vi "Button Press Event.vi"(8 "error in (no error)":errorcluster, 9 "Event Time":u32, 10 "Buttons":bool[](array[boolean]), 11 "State Data in":T1) -> (0 "error out":errorcluster, 3 "State Data out":T1)   [LabVIEW 2025]
uses:
  State Data.ctl
  Team.ctl
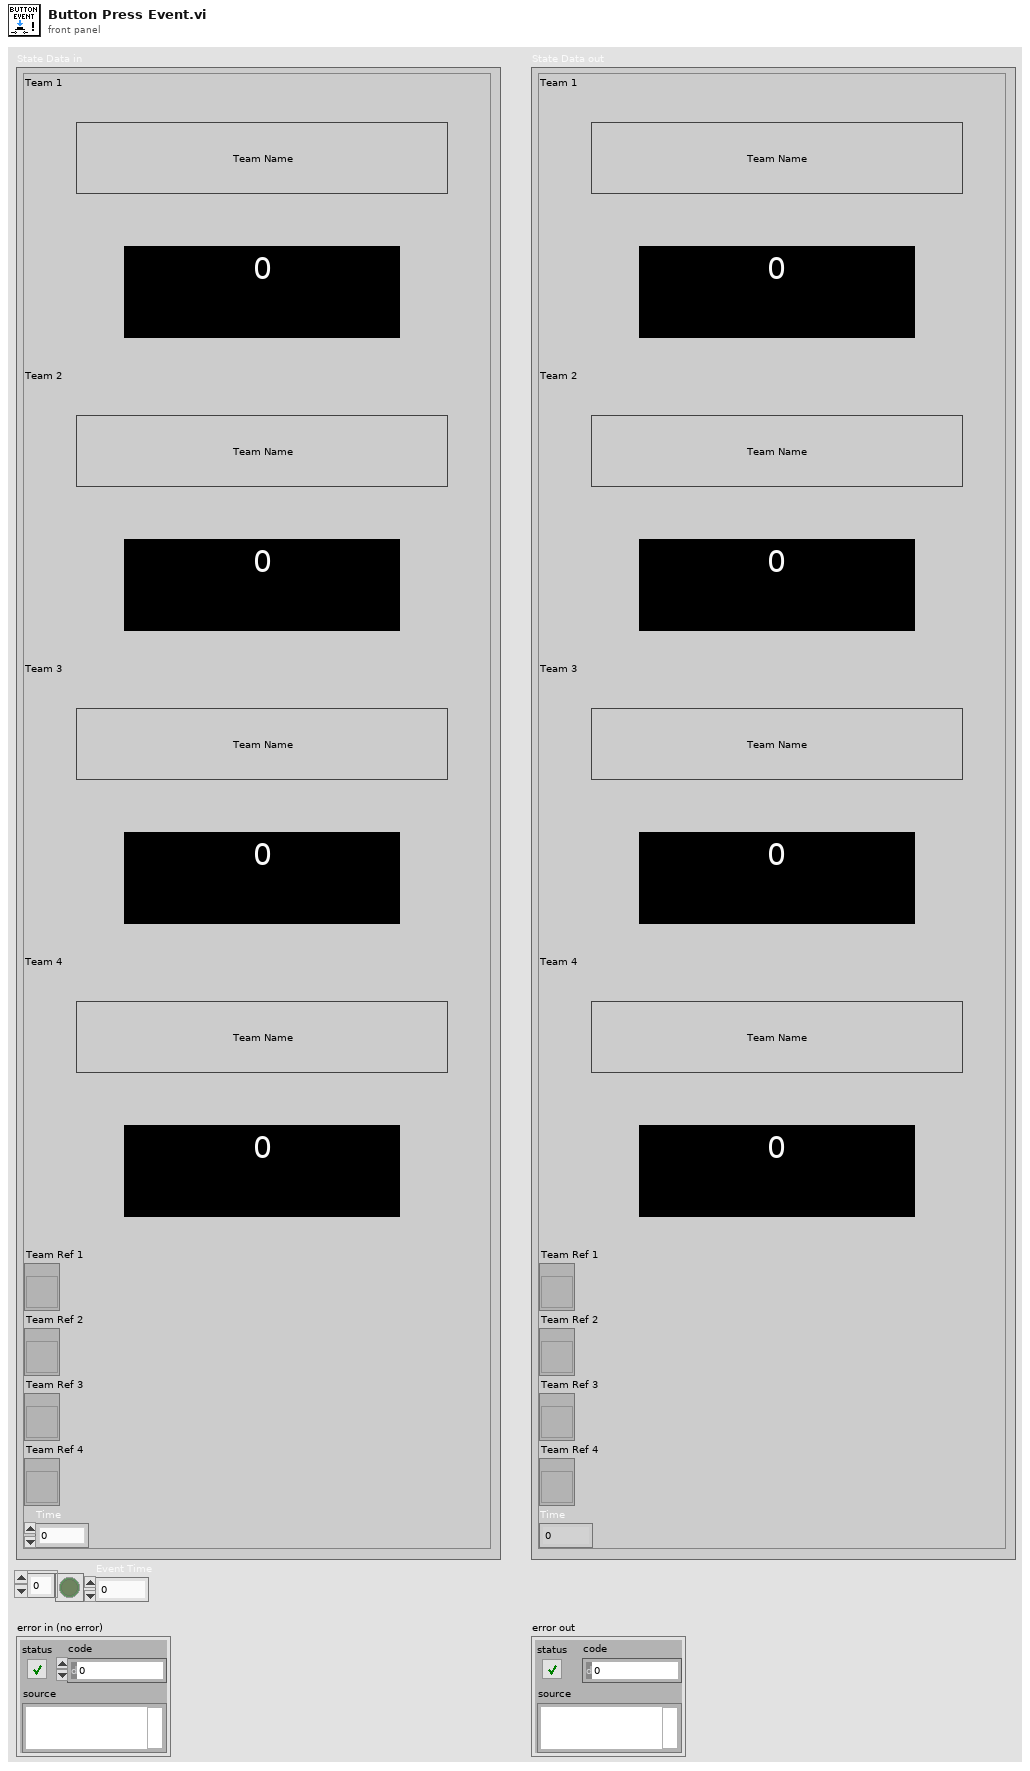
[diagram p1: front panel]
types:
  T1 = typedef "State Data.ctl" = cluster{"Team 1":T2, "Team 2":T2, "Team 3":T2, "Team 4":T2, "Team Ref 1":refnum<vi>, "Team Ref 2":refnum<vi>, "Team Ref 3":refnum<vi>, "Team Ref 4":refnum<vi>, "Time":i32}
  T2 = typedef "Team.ctl" = cluster{"ON":bool, "Name":bool, "Score":i32, "Split":string}
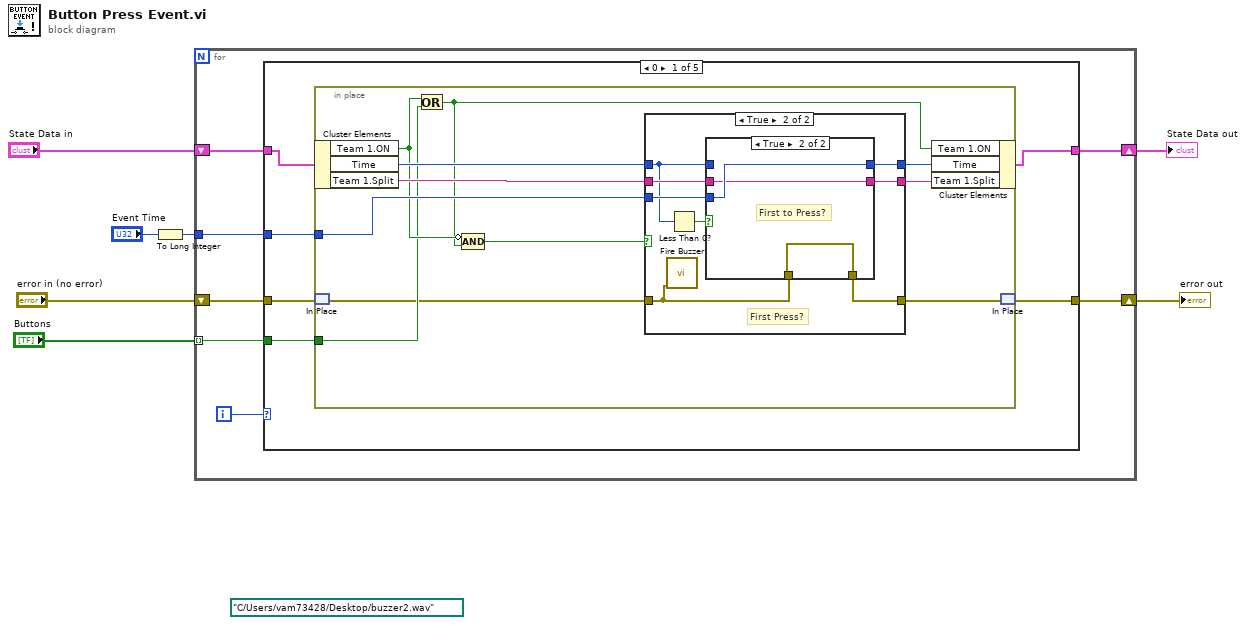
[diagram p0: block diagram]
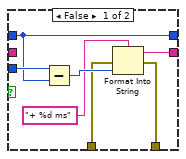
[diagram p3: hidden frame]
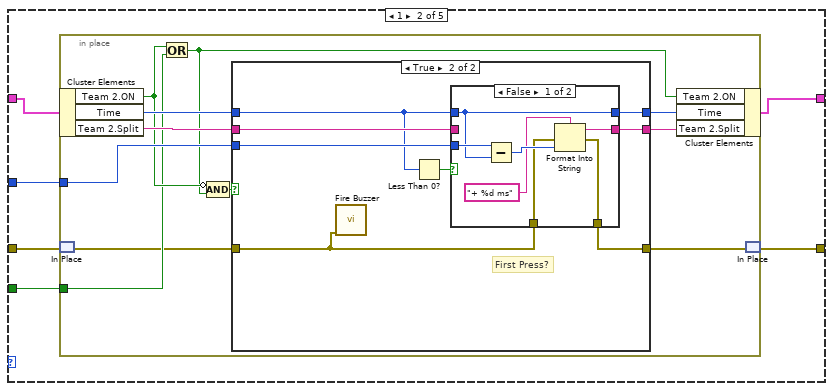
[diagram p4: hidden frame]
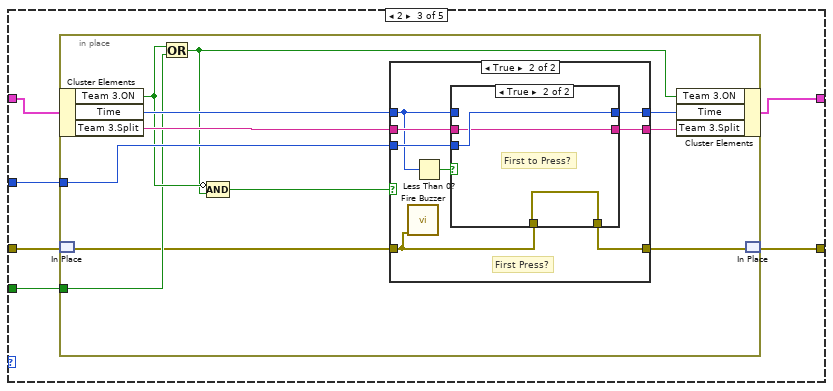
[diagram p7: hidden frame]
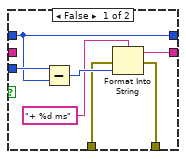
[diagram p9: hidden frame]
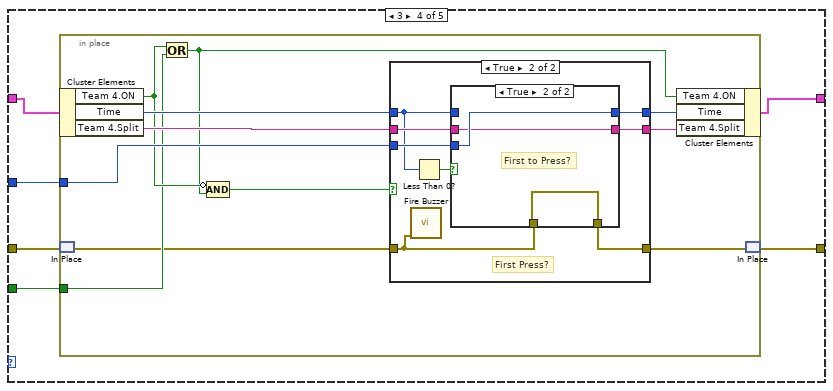
[diagram p10: hidden frame]
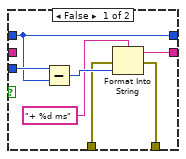
[diagram p12: hidden frame]
diagram:
  (unwired) path "C:/Users/vam73428/Desktop/buzzer2.wav" ("path")
  n1 = To Long Integer(number="Event Time") -> (32bit integer=w1:i32)
  n2 = for {
    tunnel: w1 -> [w12]
    shift-right: [w11] -> w3
    shift-left: "State Data in" -> [w13]
    tunnel: "Buttons" -> [w10] mode=indexing
    shift-right: [w8] -> w2
    shift-left: "error in (no error)" -> [w9]
    i -> [w14]
    n3 = case shown="0" w14 {
      tunnel: w13 -> [w20 w58 w96 w134 w168]
      tunnel: w12 -> [w18 w56 w94 w132 _]
      tunnel: [w15 w53 w91 w129 w168] -> w11
      tunnel: w10 -> [w19 w57 w95 w133 _]
      tunnel: w9 -> [w17 w55 w93 w131 w167]
      tunnel: [w16 w54 w92 w130 w167] -> w8
      frame 0 {
        n4 = in-place {
          in-place-border: w19 -> [w26]
          in-place-border: w18 -> [w29]
          n5 = in-place-cluster #1(w20) -> ("Team 1.ON"=w27:bool, "Time"=w31:i32, "Team 1.Split"=w30:string)
          n6 = in-place-match #2(w17) -> (w22:errorcluster)
          n7 = Or(x=w27, y=w26) -> (x .or. y?=w25:bool)
          n8 = Compound Arithmetic op=AND(invert w27, w25) -> (w24:bool)
          n9 = case shown="True" w24 {
            tunnel: w31 -> [w34 w37]
            tunnel: w30 -> [w33 w39]
            tunnel: w29 -> [_ w40]
            tunnel: [w34 w41] -> w28
            tunnel: [w33 w38] -> w23
            tunnel: w22 -> [w32 w35]
            tunnel: [w32 w36] -> w21
            frame False {
            }
            frame True {
              # "First Press?"
              n10 = call "Fire Buzzer.vi"("error in (no error)"=w35) -> ()  [unwired: 11 in]
              n11 = Less Than 0?(x=w37) -> (x < 0?=w42:bool)
              n12 = case shown="True" w42 {
                tunnel: [w45 w52] -> w41
                tunnel: w40 -> [w49 w52]
                tunnel: w39 -> [_ w51]
                tunnel: [w46 w51] -> w38
                tunnel: w37 -> [w45 _]
                tunnel: w35 -> [w44 w50]
                tunnel: [w43 w50] -> w36
                frame False {
                  n13 = Subtract(x=w49, y=w45) -> (x-y=w48:i32)
                  n14 = Format Into String(format string="+ %d ms", error in=w44, w48) -> (resulting string=w46:string, error out=w43:errorcluster)  [unwired: 1 in]
                }
                frame True {
                  # "First to Press?"
                }
              }
            }
          }
          n15 = in-place-cluster #1("Team 1.ON"=w25, "Time"=w28, "Team 1.Split"=w23) -> (w15:T1)
          n16 = in-place-match #2(w21) -> (w16:errorcluster)
        }
      }
      frame 1 {
        n17 = in-place {
          in-place-border: w57 -> [w64]
          in-place-border: w56 -> [w67]
          n18 = in-place-cluster #3(w58) -> ("Team 2.ON"=w65:bool, "Time"=w69:i32, "Team 2.Split"=w68:string)
          n19 = in-place-match #4(w55) -> (w60:errorcluster)
          n20 = Or(x=w65, y=w64) -> (x .or. y?=w63:bool)
          n21 = Compound Arithmetic op=AND(invert w65, w63) -> (w62:bool)
          n22 = case shown="True" w62 {
            tunnel: w69 -> [w72 w75]
            tunnel: w68 -> [w71 w77]
            tunnel: w67 -> [_ w78]
            tunnel: [w72 w79] -> w66
            tunnel: [w71 w76] -> w61
            tunnel: w60 -> [w70 w73]
            tunnel: [w70 w74] -> w59
            frame False {
            }
            frame True {
              # "First Press?"
              n23 = call "Fire Buzzer.vi"("error in (no error)"=w73) -> ()  [unwired: 11 in]
              n24 = Less Than 0?(x=w75) -> (x < 0?=w80:bool)
              n25 = case shown="False" w80 {
                tunnel: [w83 w90] -> w79
                tunnel: w78 -> [w87 w90]
                tunnel: w77 -> [_ w89]
                tunnel: [w84 w89] -> w76
                tunnel: w75 -> [w83 _]
                tunnel: w73 -> [w82 w88]
                tunnel: [w81 w88] -> w74
                frame False {
                  n26 = Subtract(x=w87, y=w83) -> (x-y=w86:i32)
                  n27 = Format Into String(format string="+ %d ms", error in=w82, w86) -> (resulting string=w84:string, error out=w81:errorcluster)  [unwired: 1 in]
                }
                frame True {
                  # "First to Press?"
                }
              }
            }
          }
          n28 = in-place-cluster #3("Team 2.ON"=w63, "Time"=w66, "Team 2.Split"=w61) -> (w53:T1)
          n29 = in-place-match #4(w59) -> (w54:errorcluster)
        }
      }
      frame 2 {
        n30 = in-place {
          in-place-border: w95 -> [w102]
          in-place-border: w94 -> [w105]
          n31 = in-place-cluster #5(w96) -> ("Team 3.ON"=w103:bool, "Time"=w107:i32, "Team 3.Split"=w106:string)
          n32 = in-place-match #6(w93) -> (w98:errorcluster)
          n33 = Or(x=w103, y=w102) -> (x .or. y?=w101:bool)
          n34 = Compound Arithmetic op=AND(invert w103, w101) -> (w100:bool)
          n35 = case shown="True" w100 {
            tunnel: w107 -> [w110 w113]
            tunnel: w106 -> [w109 w115]
            tunnel: w105 -> [_ w116]
            tunnel: [w110 w117] -> w104
            tunnel: [w109 w114] -> w99
            tunnel: w98 -> [w108 w111]
            tunnel: [w108 w112] -> w97
            frame False {
            }
            frame True {
              # "First Press?"
              n36 = call "Fire Buzzer.vi"("error in (no error)"=w111) -> ()  [unwired: 11 in]
              n37 = Less Than 0?(x=w113) -> (x < 0?=w118:bool)
              n38 = case shown="True" w118 {
                tunnel: [w121 w128] -> w117
                tunnel: w116 -> [w125 w128]
                tunnel: w115 -> [_ w127]
                tunnel: [w122 w127] -> w114
                tunnel: w113 -> [w121 _]
                tunnel: w111 -> [w120 w126]
                tunnel: [w119 w126] -> w112
                frame False {
                  n39 = Subtract(x=w125, y=w121) -> (x-y=w124:i32)
                  n40 = Format Into String(format string="+ %d ms", error in=w120, w124) -> (resulting string=w122:string, error out=w119:errorcluster)  [unwired: 1 in]
                }
                frame True {
                  # "First to Press?"
                }
              }
            }
          }
          n41 = in-place-cluster #5("Team 3.ON"=w101, "Time"=w104, "Team 3.Split"=w99) -> (w91:T1)
          n42 = in-place-match #6(w97) -> (w92:errorcluster)
        }
      }
      frame 3 {
        n43 = in-place {
          in-place-border: w133 -> [w140]
          in-place-border: w132 -> [w143]
          n44 = in-place-cluster #7(w134) -> ("Team 4.ON"=w141:bool, "Time"=w145:i32, "Team 4.Split"=w144:string)
          n45 = in-place-match #8(w131) -> (w136:errorcluster)
          n46 = Or(x=w141, y=w140) -> (x .or. y?=w139:bool)
          n47 = Compound Arithmetic op=AND(invert w141, w139) -> (w138:bool)
          n48 = case shown="True" w138 {
            tunnel: w145 -> [w148 w151]
            tunnel: w144 -> [w147 w153]
            tunnel: w143 -> [_ w154]
            tunnel: [w148 w155] -> w142
            tunnel: [w147 w152] -> w137
            tunnel: w136 -> [w146 w149]
            tunnel: [w146 w150] -> w135
            frame False {
            }
            frame True {
              # "First Press?"
              n49 = call "Fire Buzzer.vi"("error in (no error)"=w149) -> ()  [unwired: 11 in]
              n50 = Less Than 0?(x=w151) -> (x < 0?=w156:bool)
              n51 = case shown="True" w156 {
                tunnel: [w159 w166] -> w155
                tunnel: w154 -> [w163 w166]
                tunnel: w153 -> [_ w165]
                tunnel: [w160 w165] -> w152
                tunnel: w151 -> [w159 _]
                tunnel: w149 -> [w158 w164]
                tunnel: [w157 w164] -> w150
                frame False {
                  n52 = Subtract(x=w163, y=w159) -> (x-y=w162:i32)
                  n53 = Format Into String(format string="+ %d ms", error in=w158, w162) -> (resulting string=w160:string, error out=w157:errorcluster)  [unwired: 1 in]
                }
                frame True {
                  # "First to Press?"
                }
              }
            }
          }
          n54 = in-place-cluster #7("Team 4.ON"=w139, "Time"=w142, "Team 4.Split"=w137) -> (w129:T1)
          n55 = in-place-match #8(w135) -> (w130:errorcluster)
        }
      }
      frame Default {
      }
    }
  }
  "error out" <- w2
  "State Data out" <- w3
